vi "Update SmartRelay_Measurement in Listbox.vi"(7 "DevIDs in Config":T1[](array[typedef]), 9 "Listbox Columns":T3, 10 "SmartRelay_Measurement (Array)":T2[](array[typedef]), 11 "MulticolumnListbox in":refnum<vi>) -> ()   [LabVIEW 2018, in "EMS User Interface Actor.lvlib" / "EMS User Interface.lvclass"]
uses:
  EMS User Interface.lvclass
  Controls/Listbox Columns.ctl
  <vilib>/ORNL/CSEISMIC DDS/CSEISMIC DDS Base/Data Types/SmartRelay_Measurement.ctl
  <vilib>/ORNL/CSEISMIC DDS/CSEISMIC DDS Base/Data Types/Controls/DeviceID.ctl
  <vilib>/Utility/miscctls.llb/LVRowAndColumnTypeDef.ctl
  <vilib>/Analysis/baseanly.llb/Mean (DBL).vi
  <vilib>/Analysis/NI_AALBase.lvlib
  <vilib>/ORNL/CSEISMIC DDS/CSEISMIC DDS Base/CSEISMIC DDS.lvclass
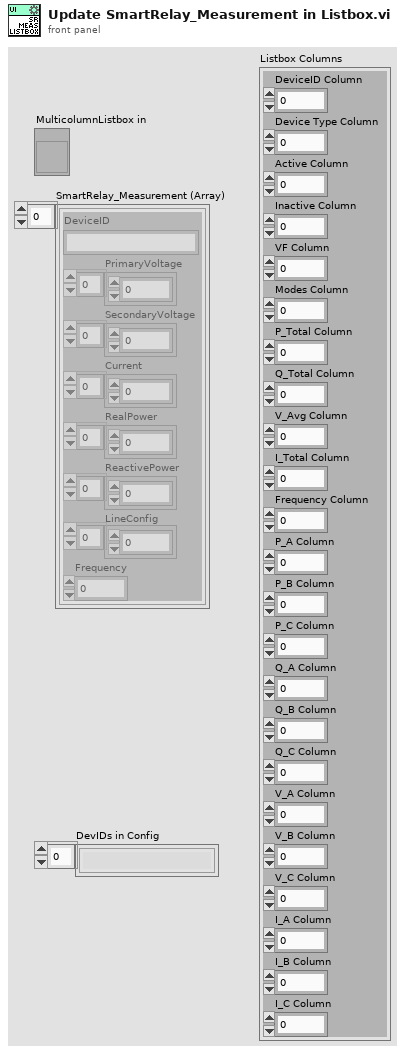
[diagram p1: front panel]
types:
  T1 = typedef "CSEISMIC DDS.lvlib/CSEISMIC DDS.lvclass/DeviceID.ctl" = string
  T2 = typedef "CSEISMIC DDS.lvlib/CSEISMIC DDS.lvclass/SmartRelay_Measurement.ctl" = cluster{"DeviceID":T1, "PrimaryVoltage":dbl[], "SecondaryVoltage":dbl[], "Current":dbl[], "RealPower":dbl[], "ReactivePower":dbl[], "LineConfig":u8[], "Frequency":dbl}
  T3 = typedef "EMS User Interface Actor.lvlib/EMS User Interface.lvclass/Listbox Columns.ctl" = cluster{"DeviceID Column":i32, "Device Type Column":i32, "Active Column":i32, "Inactive Column":i32, "VF Column":i32, "Modes Column":i32, "P_Total Column":i32, "Q_Total Column":i32, "V_Avg Column":i32, "I_Total Column":i32, "Frequency Column":i32, "P_A Column":i32, "P_B Column":i32, "P_C Column":i32, "Q_A Column":i32, "Q_B Column":i32, "Q_C Column":i32, "V_A Column":i32, "V_B Column":i32, "V_C Column":i32, "I_A Column":i32, "I_B Column":i32, "I_C Column":i32}
  T4 = typedef "LVRowAndColumnTypeDef.ctl" = cluster{"Row":i32, "Column":i32}
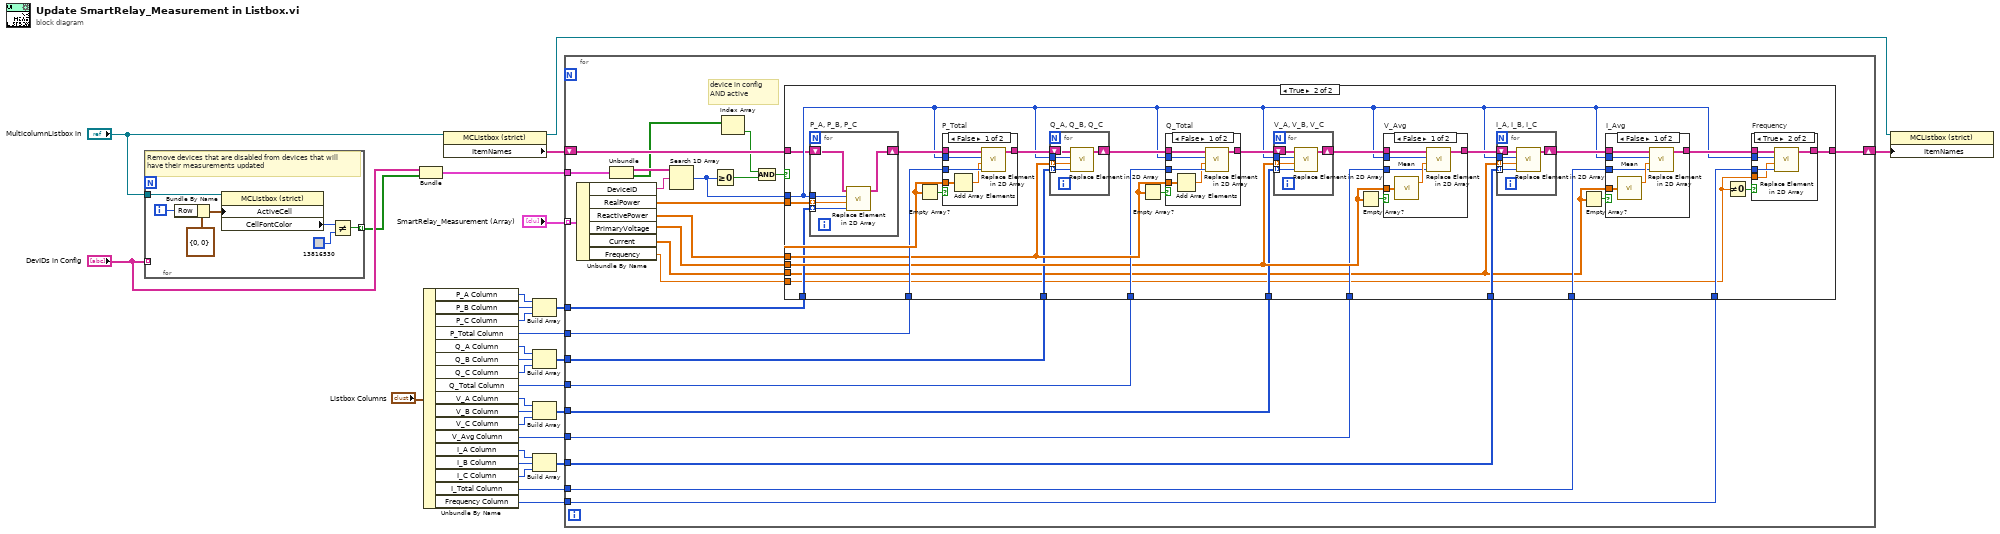
[diagram p0: block diagram]
diagram:
  n1 = for {
    tunnel: "DevIDs in Config" -> [_] mode=indexing
    tunnel: "MulticolumnListbox in" -> [w37]
    tunnel: [w31] -> w2 mode=indexing
    i -> [w34]
    # "Remove devices that are disabled from devices that will have their measurements updated"
    n2 = Bundle By Name(cluster=T4 {"Row"=0, "Column"=0} ("Active Cell:Active Cell"), "Row"=w34) -> (w35:T4)
    n3 = property on="Property Node" class="MCListbox (strict)"(reference=w37, "ActiveCell"=w35) -> ("CellFontColor"=w33:u32)  [unwired: 1 in, 2 out]
    n4 = Not Equal?(x=w33, y=u32 13816530) -> (x != y?=w31:bool)
  }
  n5 = Bundle("DevIDs in Config"="DevIDs in Config", w2) -> (w1:cluster{"DevIDs in Config":T1[], bool[]})  [unwired: 1 in]
  n6 = Unbundle By Name("Listbox Columns") -> ("P_A Column"=w26:i32, "P_B Column"=w25:i32, "P_C Column"=w24:i32, "P_Total Column"=w28:i32, "Q_A Column"=w22:i32, "Q_B Column"=w21:i32, "Q_C Column"=w20:i32, "Q_Total Column"=w27:i32, "V_A Column"=w18:i32, "V_B Column"=w17:i32, "V_C Column"=w16:i32, "V_Avg Column"=w14:i32, "I_A Column"=w13:i32, "I_B Column"=w12:i32, "I_C Column"=w11:i32, "I_Total Column"=w9:i32, "Frequency Column"=w8:i32)
  n7 = property on="Property Node" class="MCListbox (strict)"(reference="MulticolumnListbox in") -> (reference out=w5:refnum<vi>, "ItemNames"=w7:string[][])  [unwired: 1 in, 1 out]
  n8 = Build Array(w26, w25, w24) -> (w23:i32[])
  n9 = Build Array(w22, w21, w20) -> (w19:i32[])
  n10 = Build Array(w18, w17, w16) -> (w15:i32[])
  n11 = Build Array(w13, w12, w11) -> (w10:i32[])
  n12 = for {
    tunnel: w1 -> [w62]
    tunnel: "SmartRelay_Measurement (Array)" -> [w61] mode=indexing
    tunnel: w28 -> [w58]
    tunnel: w27 -> [w56]
    tunnel: w15 -> [w52]
    tunnel: w23 -> [w54]
    tunnel: w19 -> [w53]
    tunnel: w14 -> [w51]
    tunnel: w10 -> [w50]
    tunnel: w9 -> [w49]
    tunnel: w8 -> [w47]
    shift-right: [w44] -> w6
    shift-left: w7 -> [w45]
    # "device in config AND active"
    n13 = Unbundle By Name(w61) -> ("DeviceID"=w60:T1, "RealPower"=w59:dbl[], "ReactivePower"=w57:dbl[], "PrimaryVoltage"=w55:dbl[], "Current"=w48:dbl[], "Frequency"=w46:dbl)
    n14 = Unbundle(w62) -> ("DevIDs in Config"=w43:T1[], w38:bool[])
    n15 = Search 1D Array(1D array=w43, element=w60) -> (index of element=w39:i32)  [unwired: 1 in]
    n16 = Greater Or Equal To 0?(x=w39) -> (x >= 0?=w42:bool)
    n17 = Index Array(array=w38) -> (element=w41:bool)  [unwired: 1 in]
    n18 = Compound Arithmetic op=AND(w41, w42) -> (w40:bool)
    n19 = case shown="True" w40 {
      tunnel: w59 -> [_ w92]
      tunnel: w58 -> [_ w89]
      tunnel: w57 -> [_ w85]
      tunnel: w56 -> [_ w84]
      tunnel: w55 -> [_ w82]
      tunnel: w54 -> [_ w80]
      tunnel: w53 -> [_ w79]
      tunnel: w52 -> [_ w78]
      tunnel: w51 -> [_ w77]
      tunnel: w50 -> [_ w73]
      tunnel: w49 -> [_ w72]
      tunnel: w48 -> [_ w71]
      tunnel: w47 -> [_ w68]
      tunnel: w46 -> [_ w67]
      tunnel: w45 -> [w63 w65]
      tunnel: [w63 w64] -> w44
      tunnel: w39 -> [_ w69]
      frame False {
      }
      frame True {
        n20 = for "P_A, P_B, P_C" {
          tunnel: w69 -> [w104]
          tunnel: w80 -> [w100] mode=indexing
          tunnel: w92 -> [w101] mode=indexing
          shift-right: [w102] -> w93
          shift-left: w65 -> [w103]
          # "P_A, P_B, and P_C"
          n21 = call "Replace Element in 2D Array.vi"("Column"=w100, "Value"=w101, "Row"=w104, "ItemNames in"=w103) -> ("ItemNames out"=w102:string[][])  [unwired: 7 in]
        }
        n22 = Empty Array?(array=w92) -> (empty?=w91:bool)
        n23 = case "P_Total" shown="False" w91 {
          tunnel: w93 -> [w107 w111]
          tunnel: w92 -> [w110 _]
          tunnel: [w105 w111] -> w88
          tunnel: w69 -> [w106 _]
          tunnel: w89 -> [w109 _]
          frame False {
            n24 = Add Array Elements(numeric array=w110) -> (sum=w108:dbl)
            n25 = call "Replace Element in 2D Array.vi"("Column"=w109, "Value"=w108, "Row"=w106, "ItemNames in"=w107) -> ("ItemNames out"=w105:string[][])  [unwired: 7 in]
          }
          frame True {
          }
        }
        n26 = for "Q_A, Q_B, Q_C" {
          tunnel: w69 -> [w128]
          tunnel: w79 -> [w124] mode=indexing
          tunnel: w85 -> [w125] mode=indexing
          shift-right: [w126] -> w86
          shift-left: w88 -> [w127]
          # "P_A, P_B, and P_C"
          n27 = call "Replace Element in 2D Array.vi"("Column"=w124, "Value"=w125, "Row"=w128, "ItemNames in"=w127) -> ("ItemNames out"=w126:string[][])  [unwired: 7 in]
        }
        n28 = Empty Array?(array=w85) -> (empty?=w87:bool)
        n29 = case "Q_Total" shown="False" w87 {
          tunnel: w86 -> [w131 w135]
          tunnel: w85 -> [w134 _]
          tunnel: [w129 w135] -> w83
          tunnel: w69 -> [w130 _]
          tunnel: w84 -> [w133 _]
          frame False {
            n30 = Add Array Elements(numeric array=w134) -> (sum=w132:dbl)
            n31 = call "Replace Element in 2D Array.vi"("Column"=w133, "Value"=w132, "Row"=w130, "ItemNames in"=w131) -> ("ItemNames out"=w129:string[][])  [unwired: 7 in]
          }
          frame True {
          }
        }
        n32 = for "V_A, V_B, V_C" {
          tunnel: w69 -> [w140]
          tunnel: w78 -> [w136] mode=indexing
          tunnel: w82 -> [w137] mode=indexing
          shift-right: [w138] -> w81
          shift-left: w83 -> [w139]
          # "P_A, P_B, and P_C"
          n33 = call "Replace Element in 2D Array.vi"("Column"=w136, "Value"=w137, "Row"=w140, "ItemNames in"=w139) -> ("ItemNames out"=w138:string[][])  [unwired: 7 in]
        }
        n34 = Empty Array?(array=w82) -> (empty?=w90:bool)
        n35 = case "V_Avg" shown="False" w90 {
          tunnel: w81 -> [w144 w147]
          tunnel: w82 -> [w146 _]
          tunnel: [w141 w147] -> w74
          tunnel: w69 -> [w143 _]
          tunnel: w77 -> [w142 _]
          frame False {
            n36 = call-poly <vilib>:"Mean.vi"("X"=w146) -> ("mean"=w145:dbl)  [unwired: 1 out]
            n37 = call "Replace Element in 2D Array.vi"("Column"=w142, "Value"=w145, "Row"=w143, "ItemNames in"=w144) -> ("ItemNames out"=w141:string[][])  [unwired: 7 in]
          }
          frame True {
          }
        }
        n38 = for "I_A, I_B, I_C" {
          tunnel: w69 -> [w116]
          tunnel: w73 -> [w112] mode=indexing
          tunnel: w71 -> [w113] mode=indexing
          shift-right: [w114] -> w76
          shift-left: w74 -> [w115]
          # "P_A, P_B, and P_C"
          n39 = call "Replace Element in 2D Array.vi"("Column"=w112, "Value"=w113, "Row"=w116, "ItemNames in"=w115) -> ("ItemNames out"=w114:string[][])  [unwired: 7 in]
        }
        n40 = Empty Array?(array=w71) -> (empty?=w75:bool)
        n41 = case "I_Avg" shown="False" w75 {
          tunnel: w76 -> [w120 w123]
          tunnel: w71 -> [w122 _]
          tunnel: [w117 w123] -> w70
          tunnel: w69 -> [w119 _]
          tunnel: w72 -> [w118 _]
          frame False {
            n42 = call-poly <vilib>:"Mean.vi"("X"=w122) -> ("mean"=w121:dbl)  [unwired: 1 out]
            n43 = call "Replace Element in 2D Array.vi"("Column"=w118, "Value"=w121, "Row"=w119, "ItemNames in"=w120) -> ("ItemNames out"=w117:string[][])  [unwired: 7 in]
          }
          frame True {
          }
        }
        n44 = Not Equal To 0?(x=w67) -> (x != 0?=w66:bool)
        n45 = case "Frequency" shown="True" w66 {
          tunnel: w70 -> [w94 w99]
          tunnel: [w94 w98] -> w64
          tunnel: w69 -> [_ w97]
          tunnel: w68 -> [_ w96]
          tunnel: w67 -> [_ w95]
          frame False {
          }
          frame True {
            n46 = call "Replace Element in 2D Array.vi"("Column"=w96, "Value"=w95, "Row"=w97, "ItemNames in"=w99) -> ("ItemNames out"=w98:string[][])  [unwired: 7 in]
          }
        }
      }
    }
  }
  n47 = property on="Property Node" class="MCListbox (strict)"(reference=w5, "ItemNames"=w6) -> ()  [unwired: 1 in, 2 out]
